vi "Nearest Setpoint.vi"(8 "error in (no error)":errorcluster, 10 "Encoder":dbl, 11 "Direction":T2) -> (0 "error out":errorcluster, 2 "State":T1, 3 "Setpoint":dbl)   [LabVIEW 2014]
doc: "Determines the nearest setpoint for the PID when switching from manual mode.\n\n<b>Setpoints</b> - a decreasing array of setpoints (i.e. 0, -100, -500, -2000)"
uses:
  Elevator Direction.ctl
  Elevator States.ctl
  Elevator Setpoints.ctl
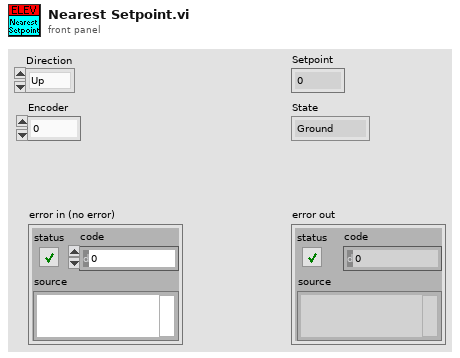
[diagram p1: front panel]
types:
  T1 = typedef "Elevator States.ctl" = enum16{"Ground", "Tote 1", "Tote 2", "Tote 3", "Tote 4", "Tote 5", "Tote 6"}
  T2 = typedef "Elevator Direction.ctl" = enum16{"Up", "Down"}
  T3 = typedef "Elevator Setpoints.ctl" = dbl[]
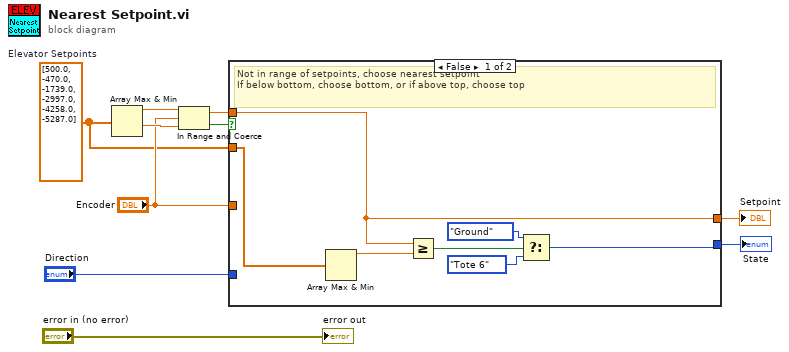
[diagram p0: block diagram]
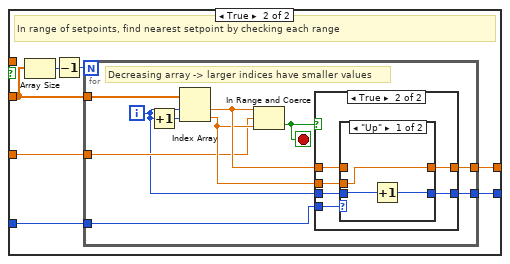
[diagram p2: hidden frame]
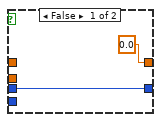
[diagram p3: hidden frame]
diagram:
  w3 = T3 [500.0, -470.0, -1739.0, -2997.0, -4258.0, -5287.0]  # Elevator Setpoints
  n1 = Array Max & Min(array=w3) -> (max value=w8:dbl, min value=w7:dbl)  [unwired: 2 out]
  n2 = In Range and Coerce(upper limit=w8, x="Encoder", lower limit=w7) -> (coerced(x)=w4:dbl, In Range?=w6:bool)
  n3 = case shown="False" w6 {
    tunnel: "Direction" -> [_ w23]
    tunnel: [w15 w22] -> w9
    tunnel: w3 -> [w17 w21]
    tunnel: "Encoder" -> [_ w20]
    tunnel: w4 -> [w15 _]
    tunnel: [w11 w18] -> w1
    frame False {
      # "Not in range of setpoints, choose nearest setpoint\nIf below bottom, choose bottom, or if above top, choose top"
      n4 = Array Max & Min(array=w17) -> (max value=w16:dbl)  [unwired: 3 out]
      n5 = Greater Or Equal?(x=w15, y=w16) -> (x >= y?=w14:bool)
      n6 = Select(t=Elevator_States."Ground" ("Enum"), s=w14, f=Elevator_States."Tote 6" ("Enum")) -> (s? t:f=w11:T1)
    }
    frame True {
      # "In range of setpoints, find nearest setpoint by checking each range"
      n7 = Array Size(array=w21) -> (size(s)=w24:i32)
      n8 = Decrement(x=w24) -> (x-1=w19:i32)
      n9 = for {
        N: w19 -> [_]
        tunnel: w21 -> [w33]
        tunnel: w23 -> [w31]
        tunnel: [w28] -> w22
        tunnel: w20 -> [w27]
        tunnel: [w25] -> w18
        i -> [w26]
        stop <- w32 stop-if-true
        # "Decreasing array -> larger indices have smaller values"
        n10 = Increment(x=w26) -> (x+1=w34:i32)
        n11 = Index Array(array=w33, index #1=w26, index #2=w34) -> (element #1=w30:dbl, element #2=w29:dbl)
        n12 = In Range and Coerce(upper limit=w30, x=w27, lower limit=w29) -> (In Range?=w32:bool)  [unwired: 1 out]
        n13 = case shown="True" w32 {
          tunnel: w31 -> [_ w42]
          tunnel: w30 -> [_ w41]
          tunnel: w29 -> [_ w40]
          tunnel: [0.0 w39] -> w28
          tunnel: w26 -> [w35 w38]
          tunnel: [w35 w37] -> w25
          frame False {
          }
          frame True {
            n14 = case shown="\"Up\"" w42 {
              tunnel: [w45 w47] -> w39
              tunnel: w41 -> [_ w47]
              tunnel: w40 -> [w45 _]
              tunnel: w38 -> [w44 w46]
              tunnel: [w43 w46] -> w37
              frame "Up" {
                n15 = Increment(x=w44) -> (x+1=w43:i32)
              }
              frame "Down" {
              }
            }
          }
        }
      }
    }
  }
  "Setpoint" <- w9
  "State" <- w1
  "error out" <- "error in (no error)"
